vi "適應性控制_多頻率追蹤_V3(電腦模擬).vi"() -> ()   [LabVIEW 2010]
panel:
  in  "理想初始頻率(Hz)":dbl=1.0
  in  "理想頻率數":i32=10
  out "權重":dbl[](graph)
  out "當下誤差":dbl=0.1 format="%#_13g"
  out "模擬輸入x(t)":dbl[](graph)
  in  "頻率間距":dbl=1.0
  out "理想與FIR輸出":dbl[][](graph)
  out "message":string=" INSTRUCTIONS:\r\rNormal Use:  When using subVIs that incorporate the error in/error out (or error I/O) structure, place this handler where you want to inform the user of an error, typically at the end of the I/O data path, as the last action of the program.  If the error in error? is ERROR, the handler creates a message describing the error and its source.  If the type of dialog = 1 (default), the message is displayed to the user, who can only acknowedge it.  If the type = 2, the user can acknowledge the message or abort execution; aborting a program with active I/O is not recommended.  If the type = 0, no message is displayed; this is used to process the error programmatically, and the error out cluster elements are wired to individual terminals for that reason.  \r\rOther Use:\n\r\nlocal testing.  To test the error code of a subVI or function that does not have the error I/O structure, you can wire its error code and a source string to the local error code and error source inputs.  If error in error? indicates no error and error code is not equal to 0, the local code and source are substituted for the error in values, and error? is set TRUE (ERROR)."
  out "誤差":dbl(graph)
  out "while平均運行時間":dbl
  out "收斂time":dbl
  out "各頻率誤差已達標準":bool
  in  "各頻率誤差低於多少亮燈":dbl=0.1 format="%#_13g"
  out "權重(w)":dbl[](array[numeric])
  in  "理想振幅":dbl=1.0
  in  "理想直流偏移":dbl
  in  "理想相位(deg)":dbl
  in  "收斂係數":dbl=0.0001
  in  "頻率數":i32=10
  in  "order":i32=100
  in  "模擬相位(deg)":dbl
  in  "初始頻率(Hz)":dbl=1.0
  in  "取樣頻率":dbl=100.0 min=1.0 max=1000.0 step=1.0
  in  "模擬直流偏移":dbl
  in  "模擬振幅振幅":dbl=1.0
  in  "stop":bool
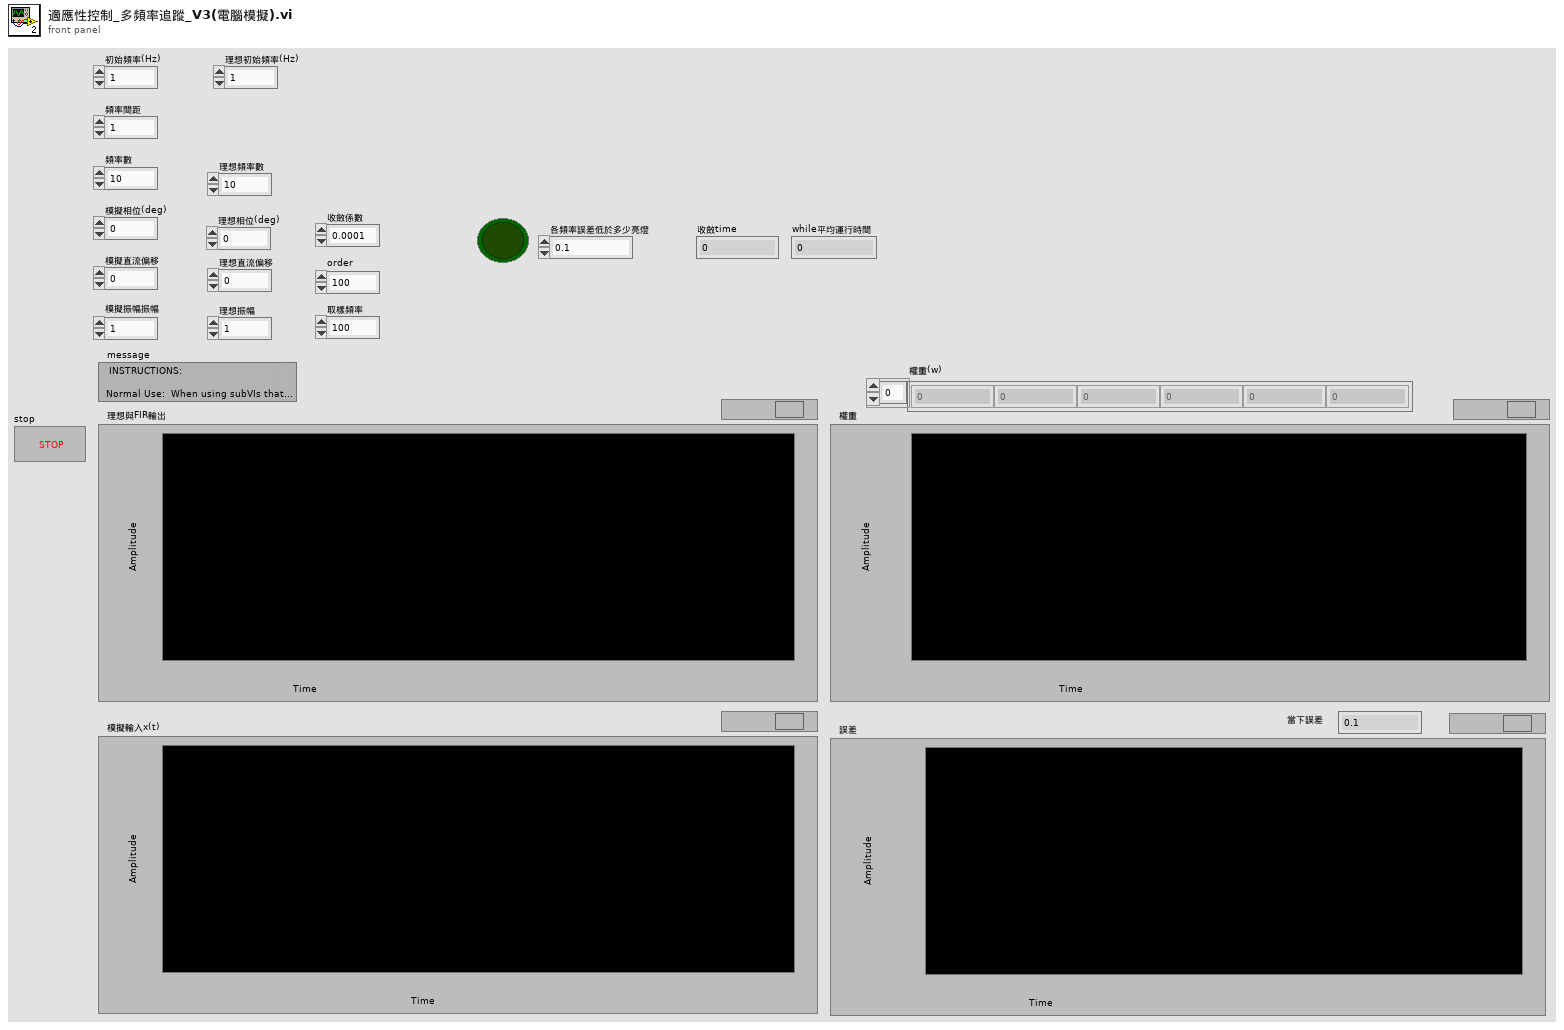
[diagram p1: front panel]
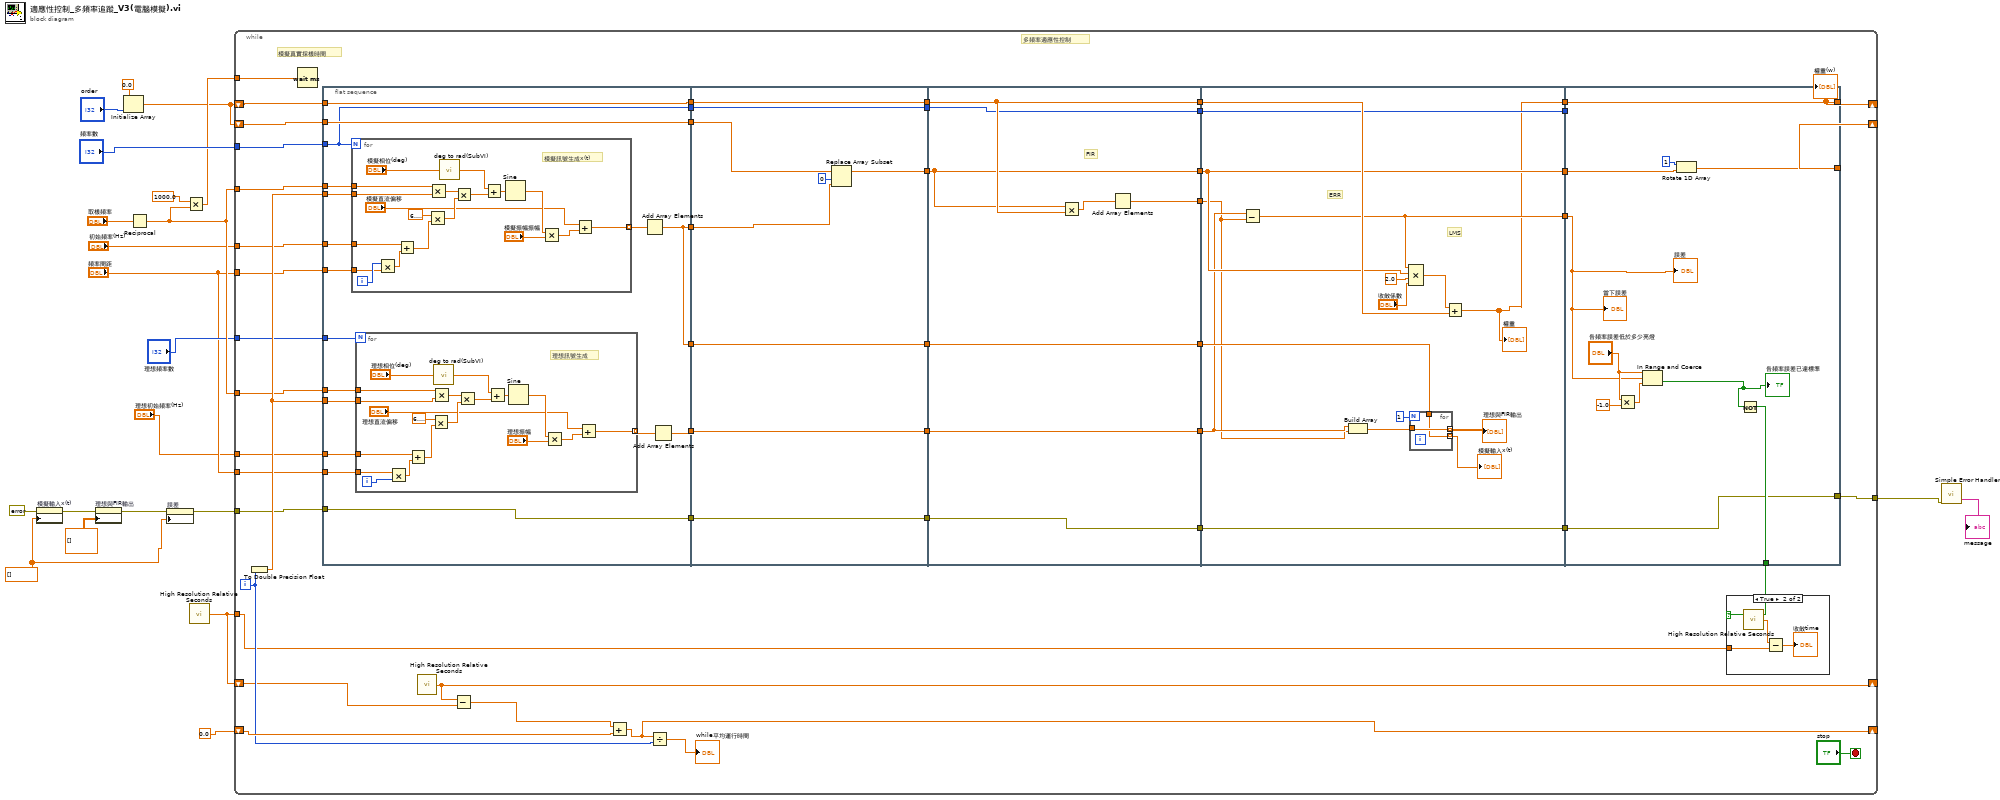
[diagram p0: block diagram]
diagram:
  w5 = dbl[] [] ("History Data")
  n1 = property on="模擬輸入x(t)" class="WFChart (strict)"(error in=errorcluster {"status"=FALSE, "code"=0, "source"=""} ("error constant"), "History Data"=w5) -> (error out=w9:errorcluster)  [unwired: 1 in, 1 out]
  n2 = property on="理想與FIR輸出" class="WFChart (strict)"(error in=w9, "History Data"=dbl[][] []) -> (error out=w10:errorcluster)  [unwired: 1 in, 1 out]
  n3 = Initialize Array(0.0 ("element"), "order") -> (w4:dbl[])
  n4 = Reciprocal(x="取樣頻率") -> (1/x=w19:dbl)
  n5 = property on="誤差" class="WFChart (strict)"(error in=w10, "History Data"=w5) -> (error out=w12:errorcluster)  [unwired: 1 in, 1 out]
  n6 = Multiply(x=1000.0, y=w19) -> (x*y=w17:dbl)
  n7 = call <vilib>:"High Resolution Relative Seconds.vi"() -> ("relative seconds"=w16:dbl)
  n8 = while {
    tunnel: "頻率數" -> [w70]
    shift-right: [w26] -> _
    shift-left: w4 -> [w71]
    shift-right: [w55] -> _
    shift-left: w4 -> [w63]
    tunnel: w19 -> [w50]
    tunnel: w19 -> [w49]
    tunnel: w17 -> [w39]
    tunnel: w16 -> [w41]
    shift-right: [w42] -> _
    shift-left: w16 -> [w40]
    shift-right: [w43] -> _
    shift-left: 0.0 -> [w45]
    tunnel: "初始頻率(Hz)" -> [w37]
    tunnel: [w36] -> w13
    tunnel: w12 -> [w31]
    tunnel: "頻率間距" -> [w30]
    tunnel: "理想頻率數" -> [w25]
    tunnel: "頻率間距" -> [w24]
    tunnel: "理想初始頻率(Hz)" -> [w23]
    i -> [w44]
    stop <- "stop" stop-if-true
    # "模擬真實採樣時間"
    # "多頻率適應性控制"
    n9 = To Double Precision Float(number=w44) -> (double precision float=w61:dbl)
    n10 = Wait (ms)(milliseconds to wait=w39) -> ()  [unwired: 1 out]
    n11 = flat-sequence {
      tunnel: w61 -> [w93]
      tunnel: [w92] -> w72
      tunnel: w71 -> [w92]
      tunnel: w70 -> [w90]
      tunnel: [w82] -> w69
      tunnel: [w90] -> w68
      tunnel: [w91] -> w64
      tunnel: w63 -> [w91]
      tunnel: w61 -> [w89]
      tunnel: [w77] -> w58
      tunnel: w50 -> [w88]
      tunnel: w49 -> [w87]
      tunnel: w37 -> [w86]
      tunnel: [w85] -> w32
      tunnel: w31 -> [w85]
      tunnel: w30 -> [w84]
      tunnel: [w82] -> w27
      tunnel: w25 -> [w81]
      tunnel: w24 -> [w80]
      tunnel: w23 -> [w79]
      tunnel: w72 -> [w136]
      tunnel: w69 -> [w135]
      tunnel: w68 -> [w140]
      tunnel: [w140] -> w67
      tunnel: [w139] -> w66
      tunnel: [w138] -> w65
      tunnel: w64 -> [w138]
      tunnel: [w137] -> w59
      tunnel: w58 -> [w137]
      tunnel: [w134] -> w33
      tunnel: w32 -> [w134]
      tunnel: [w133] -> w28
      tunnel: w27 -> [w133]
      tunnel: w67 -> [w145]
      tunnel: w66 -> [w141]
      tunnel: w65 -> [w148]
      tunnel: [w148] -> w62
      tunnel: [w147] -> w60
      tunnel: w59 -> [w147]
      tunnel: [w146] -> w57
      tunnel: [w141] -> w56
      tunnel: [w145] -> w52
      tunnel: [w144] -> w34
      tunnel: w33 -> [w144]
      tunnel: [w143] -> w29
      tunnel: w28 -> [w143]
      tunnel: w62 -> [w164]
      tunnel: w60 -> [w150]
      tunnel: w57 -> [w149]
      tunnel: w56 -> [w154]
      tunnel: [w151] -> w54
      tunnel: [w161] -> w53
      tunnel: w52 -> [w161]
      tunnel: [w154] -> w51
      tunnel: [w155] -> w48
      tunnel: [w160] -> w35
      tunnel: w34 -> [w160]
      tunnel: w29 -> [w159]
      tunnel: [w177] -> w55
      tunnel: w54 -> [w177]
      tunnel: w53 -> [_]
      tunnel: w51 -> [w169]
      tunnel: [w176] -> w26
      tunnel: w48 -> [w167]
      tunnel: [w172] -> w38
      tunnel: [w171] -> w36
      tunnel: w35 -> [w171]
      frame #0 {
        n12 = for {
          N: w90 -> [_]
          tunnel: w93 -> [w121]
          tunnel: [w118] -> w83 mode=indexing
          tunnel: w88 -> [w117]
          tunnel: w86 -> [w116]
          tunnel: w84 -> [w114]
          i -> [w115]
          # "模擬訊號生成x(t)"
          n13 = Multiply(x=w115, y=w114) -> (x*y=w113:dbl)
          n14 = Add(x=w116, y=w113) -> (x+y=w119:dbl)
          n15 = Multiply(x=6.283185307179586, y=w119) -> (x*y=w129:dbl)
          n16 = Multiply(x=w117, y=w121) -> (x*y=w122:dbl)
          n17 = call "deg to rad(SubVI).vi"("Degree"="模擬相位(deg)") -> ("Radian"=w126:dbl)
          n18 = Multiply(x=w122, y=w129) -> (x*y=w130:dbl)
          n19 = Add(x=w126, y=w130) -> (x+y=w131:dbl)
          n20 = Sine(x=w131) -> (sin(x)=w127:dbl)
          n21 = Multiply(x=w127, y="模擬振幅振幅") -> (x*y=w128:dbl)
          n22 = Add(x="模擬直流偏移", y=w128) -> (x+y=w118:dbl)
        }
        n23 = for {
          N: w81 -> [_]
          tunnel: w89 -> [w112]
          tunnel: [w111] -> w78 mode=indexing
          tunnel: w87 -> [w110]
          tunnel: w80 -> [w96]
          tunnel: w79 -> [w95]
          i -> [w97]
          # "理想訊號生成"
          n24 = Multiply(x=w96, y=w97) -> (x*y=w98:dbl)
          n25 = Add(x=w95, y=w98) -> (x+y=w94:dbl)
          n26 = Multiply(x=6.283185307179586, y=w94) -> (x*y=w107:dbl)
          n27 = Multiply(x=w110, y=w112) -> (x*y=w100:dbl)
          n28 = call "deg to rad(SubVI).vi"("Degree"="理想相位(deg)") -> ("Radian"=w104:dbl)
          n29 = Multiply(x=w100, y=w107) -> (x*y=w108:dbl)
          n30 = Add(x=w104, y=w108) -> (x+y=w109:dbl)
          n31 = Sine(x=w109) -> (sin(x)=w105:dbl)
          n32 = Multiply(x=w105, y="理想振幅") -> (x*y=w106:dbl)
          n33 = Add(x="理想直流偏移", y=w106) -> (x+y=w111:dbl)
        }
        n34 = Add Array Elements(numeric array=w83) -> (sum=w82:dbl)
        n35 = Add Array Elements(numeric array=w78) -> (sum=w77:dbl)
      }
      frame #1 {
        n36 = Replace Array Subset(array=w136, new element=w135, index=0) -> (w139:dbl[])
      }
      frame #2 {
        # "FIR"
        n37 = Multiply(x=w141, y=w148) -> (x*y=w142:dbl[])
        n38 = Add Array Elements(numeric array=w142) -> (sum=w146:dbl)
      }
      frame #3 {
        # "LMS"
        # "ERR"
        n39 = Subtract(x=w150, y=w149) -> (x-y=w155:dbl)
        n40 = Build Array(w150, w149) -> (w162:dbl[])
        n41 = Compound Arithmetic op=MULTIPLY(w155, w154, 2.0, "收斂係數") -> (w153:dbl[])
        n42 = for {
          N: 1 -> [_]
          tunnel: [w166] -> w152 mode=indexing
          tunnel: w162 -> [w166]
          tunnel: [w165] -> w158 mode=indexing
          tunnel: w159 -> [w165]
        }
        "理想與FIR輸出" <- w152
        "模擬輸入x(t)" <- w158
        n43 = Add(x=w153, y=w164) -> (x+y=w151:dbl[])
        "權重" <- w151
      }
      frame #4 {
        n44 = Multiply(x="各頻率誤差低於多少亮燈", y=-1.0) -> (x*y=w173:dbl)
        n45 = In Range and Coerce(upper limit="各頻率誤差低於多少亮燈", x=w167, lower limit=w173) -> (In Range?=w168:bool)  [unwired: 1 out]
        "各頻率誤差已達標準" <- w168
        n46 = Rotate 1D Array(1:w169, 2:1 ("n")) -> (0:w176:dbl[])
        n47 = Not(x=w168) -> (.not. x?=w172:bool)
        "誤差" <- w167
        "當下誤差" <- w167
      }
    }
    n48 = call <vilib>:"High Resolution Relative Seconds.vi"() -> ("relative seconds"=w42:dbl)
    n49 = Subtract(x=w42, y=w40) -> (x-y=w47:dbl)
    n50 = Add(x=w47, y=w45) -> (x+y=w43:dbl)
    n51 = Divide(x=w43, y=w44) -> (x/y=→"while平均運行時間":dbl)
    n52 = case shown="True" w38 {
      tunnel: w41 -> [_ w74]
      frame False {
      }
      frame True {
        n53 = call <vilib>:"High Resolution Relative Seconds.vi"() -> ("relative seconds"=w76:dbl)
        n54 = Subtract(x=w76, y=w74) -> (x-y=→"收斂time":dbl)
      }
    }
    "權重(w)" <- w55
  }
  n55 = call <vilib>:"Simple Error Handler.vi"("error in (no error)"=w13) -> ("message"=→"message":string)  [unwired: 4 in, 4 out]
